vi "Write #cars owned.vi"(8 "error in (no error)":errorcluster, 10 "#cars owned":i16, 11 "Michael Jordan in":refnum<class "Michael Jordan.lvclass">) -> (0 "error out":errorcluster, 3 "Michael Jordan out":refnum<class "Michael Jordan.lvclass">)   [LabVIEW 2019, in "Michael Jordan.lvclass"]
uses:
  Michael Jordan.lvclass
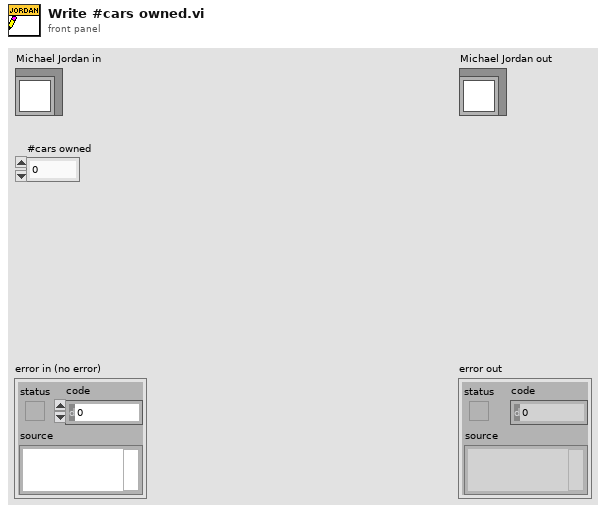
[diagram p1: front panel]
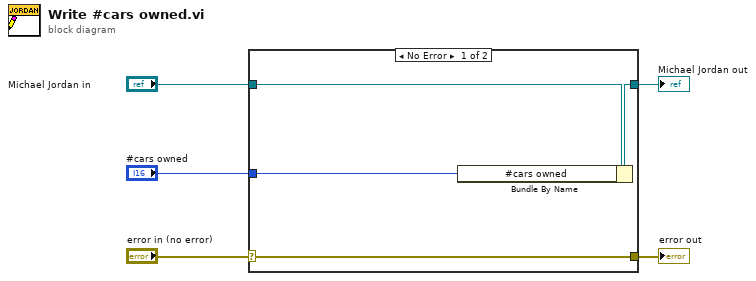
[diagram p0: block diagram]
diagram:
  n1 = case shown="No Error" "error in (no error)" {
    selector: "error in (no error)" -> [w9 w10]
    tunnel: [w9 w10] -> w4
    tunnel: [w7 w11] -> w2
    tunnel: "Michael Jordan in" -> [w8 w11]
    tunnel: "#cars owned" -> [w6 _]
    frame No Error {
      n2 = Bundle By Name(cluster=w8, "#cars owned"=w6) -> (w7:refnum<class "Michael Jordan.lvclass">)
    }
    frame Error {
    }
  }
  "error out" <- w4
  "Michael Jordan out" <- w2
